vi "PathCal.vi"(9 "pose_y":dbl=7988.0, 10 "pose_x":dbl=8250.0, 11 "语音命令数组":string[][](array[string])) -> (2 "Local_Goal":T1, 3 "Goal_Path":dbl[][](array[numeric]))   [LabVIEW 2014]
uses:
  ctl/Point.ctl
panel:
  out "Path 2":string[](array[string])
  out "Area 3":string[](array[string])
  out "Dis 2":dbl
  out "Path坐标数组":dbl[][](array[numeric])
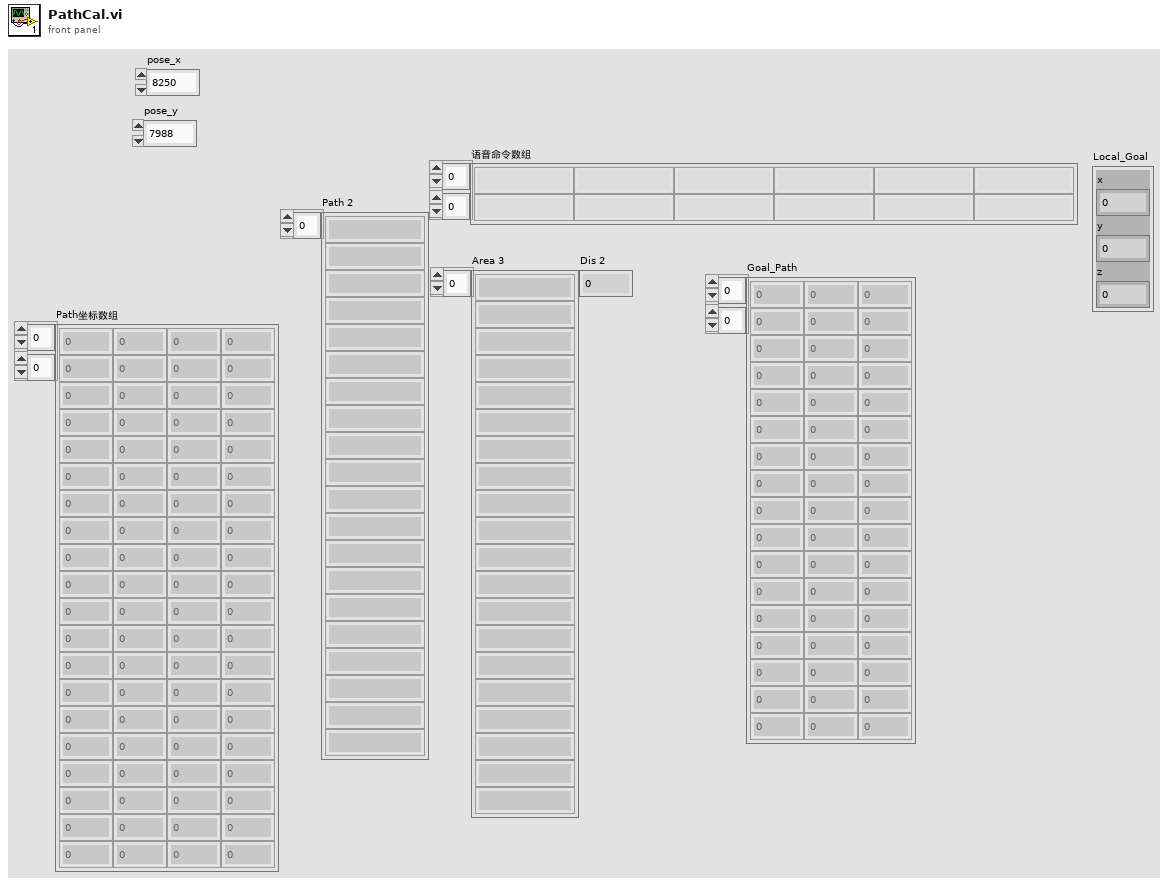
[diagram p1: front panel]
types:
  T1 = typedef "Point.ctl" = cluster{"x":dbl, "y":dbl, "z":dbl}
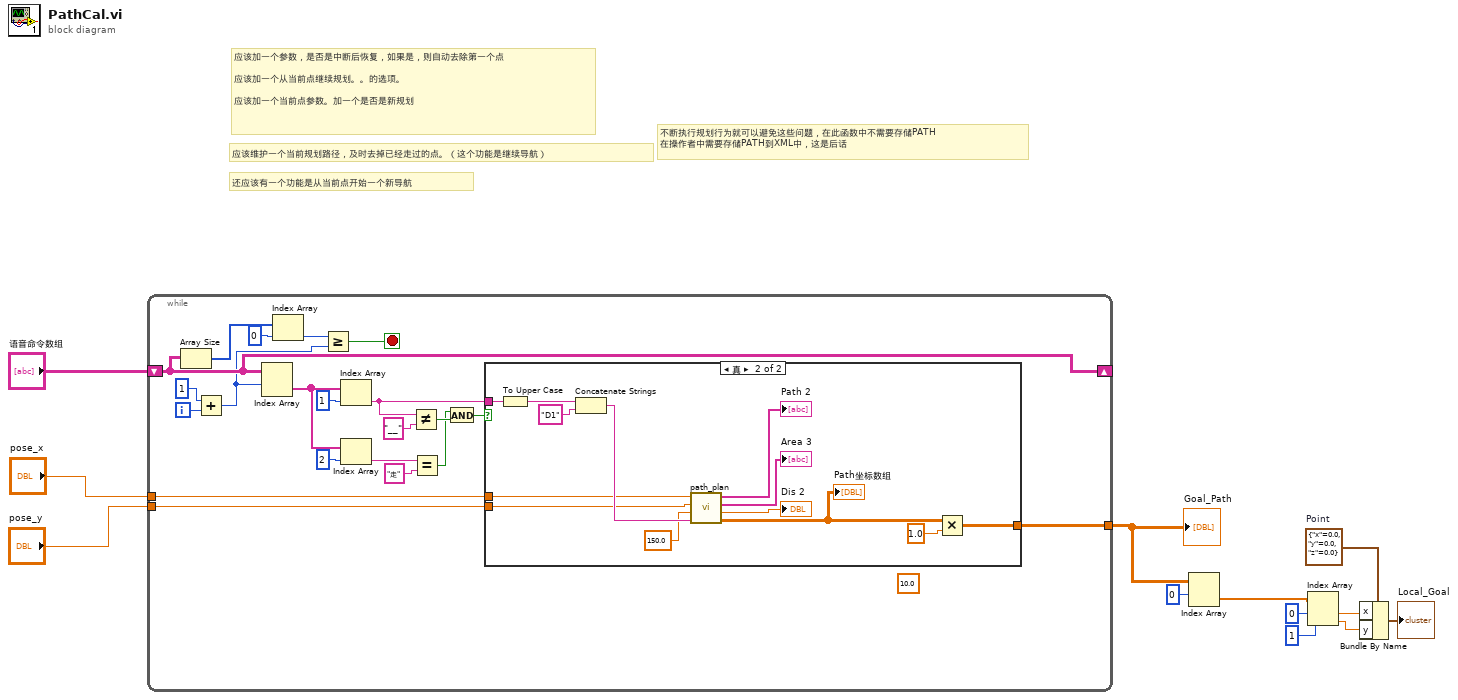
[diagram p0: block diagram]
diagram:
  w2 = T1 {"x"=0.0, "y"=0.0, "z"=0.0}  # Point
  # "不断执行规划行为就可以避免这些问题，在此函数中不需要存储PATH\n在操作者中需要存储PATH到XML中，这是后话"
  # "还应该有一个功能是从当前点开始一个新导航"
  # "应该维护一个当前规划路径，及时去掉已经走过的点。（这个功能是继续导航）"
  # "应该加一个参数，是否是中断后恢复，如果是，则自动去除第一个点\n\n应该加一个从当前点继续规划。。的选项。\n\n应该加一个当前点参数。加一个是否是新规划"
  n1 = while {
    shift-right: [w29] -> _
    shift-left: "语音命令数组" -> [w29]
    tunnel: [w15] -> w9
    tunnel: "pose_x" -> [w14]
    tunnel: "pose_y" -> [w13]
    i -> [w31]
    stop <- w28 stop-if-true
    (unwired) 10.0
    n2 = Array Size(array=w29) -> (size(s)=w33:i32[])
    n3 = Add(x=1, y=w31) -> (x+y=w26:i32)
    n4 = Index Array(array=w29, index (row)=w26) -> (element=w21:string[])  [unwired: 1 in]
    n5 = Index Array(array=w33, index=0 ("索引")) -> (element=w27:i32)
    n6 = Greater Or Equal?(x=w27, y=w26) -> (x >= y?=w28:bool)
    n7 = Index Array(array=w21, index=1 ("索引")) -> (element=w16:string)
    n8 = Index Array(array=w21, index=2 ("索引")) -> (element=w24:string)
    n9 = Not Equal?(x=w16, y="__") -> (x != y?=w19:bool)
    n10 = Equal?(x=w24, y="走") -> (x = y?=w18:bool)
    n11 = And(x=w18, y=w19) -> (x .and. y?=w17:bool)
    n12 = case shown="真" w17 {
      tunnel: w16 -> [_ w46]
      tunnel: [_ w37] -> w15
      tunnel: w14 -> [_ w35]
      tunnel: w13 -> [_ w34]
      frame False {
      }
      frame True {
        n13 = To Upper Case(1:w46) -> (0:w45:string)
        n14 = Concatenate Strings(w45, "D1" ("字符串")) -> (w43:string)
        n15 = call "path_plan.vi"("Node2"=w43, "z"=150.0, "y"=w34, "x"=w35) -> ("Path坐标数组"=w38:dbl[][], "Dis 2"=→"Dis 2":dbl, "Area 3"=→"Area 3":string[], "Path 2"=→"Path 2":string[])
        "Path坐标数组" <- w38
        n16 = Multiply(x=w38, y=1.0) -> (x*y=w37:dbl[][])
      }
    }
  }
  "Goal_Path" <- w9
  n17 = Index Array(array=w9, index (row)=0 ("索引 (行)")) -> (element=w7:dbl[])  [unwired: 1 in]
  n18 = Index Array(array=w7, index #1=0 ("索引"), index #2=1 ("索引")) -> (element #1=w4:dbl, element #2=w3:dbl)
  n19 = Bundle By Name(cluster=w2, "x"=w4, "y"=w3) -> (→"Local_Goal":T1)
